vi "Read As File_Sync.vi"(7 "mode (OpenOrCreate)":i32(ring)=4 items=["CreateNew"=1, "Create"=2, "Open"=3, "OpenOrCreate"=4, "Truncate"=5, "Append"=6], 8 "error in (no error)":errorcluster, 10 "FilePath":path, 11 "HttpContent in":refnum<class "HttpContent.lvclass">) -> (0 "error out":errorcluster, 1 "IsCompleted":bool, 2 "FilePath (dup)":path, 3 "HttpContent out":refnum<class "HttpContent.lvclass">, 4 "Canceled":bool)   [LabVIEW 2018, in "HttpClient_NET.lvlib" / "HttpContent.lvclass"]
doc: "<b> </b> <b> </b>\nHttpClient_NET\nJustin Young - Viviota\nCopyright (c) 2021\nLicense: BSD"
uses:
  HttpContent.lvclass
  Types/HttpNet_error_enum.ctl
  HttpClient_NET.lvlib
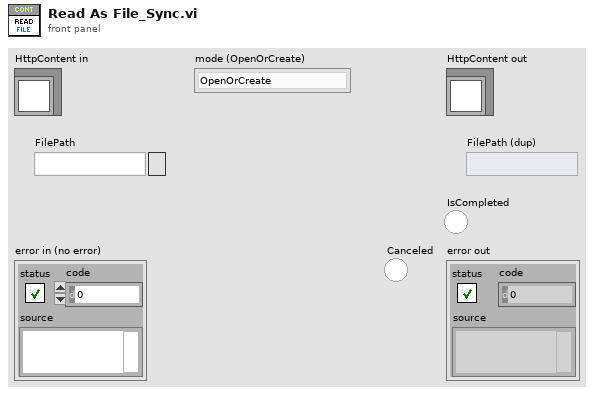
[diagram p1: front panel]
types:
  T1 = typedef "HttpClient_NET.lvlib/HttpNet_error_enum.ctl" = enum16{"REST method is not available", "URL cannot be blank", "Output filepath cannot be empty", "Input filepath cannot be empty", "Internal .NET error %s", "Output filepath cannot be directory", "Download Task no longer exists", "Mutipart Put not supported from REST Client Interface.  Please revert to lower level classes"}
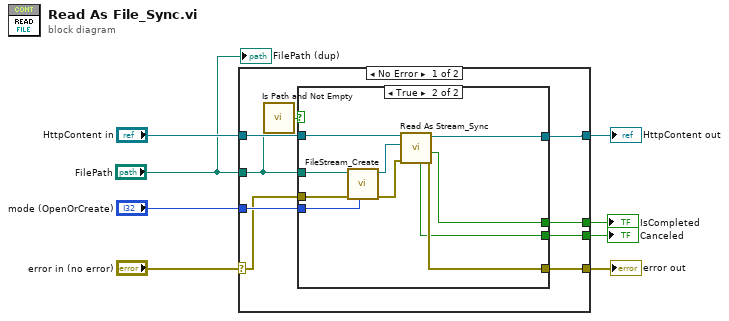
[diagram p0: block diagram]
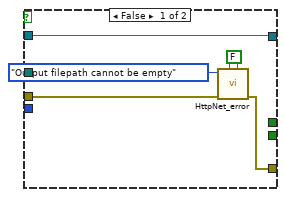
[diagram p2: hidden frame]
diagram:
  n1 = case shown="No Error" "error in (no error)" {
    selector: "error in (no error)" -> [w13 w34]
    tunnel: [w14 w34] -> w7
    tunnel: [w16 w33] -> w5
    tunnel: "HttpContent in" -> [w17 w33]
    tunnel: "mode (OpenOrCreate)" -> [w15 _]
    tunnel: "FilePath" -> [w10 _]
    tunnel: [w12 _] -> w2
    tunnel: [w11 _] -> w1
    frame No Error {
      n2 = call <vilib>:"Is Path and Not Empty.vi"("path"=w10) -> ("Is Path and Not Empty?"=w9:bool)  [unwired: 4 in]
      n3 = case shown="True" w9 {
        tunnel: w17 -> [w22 w32]
        tunnel: [w22 w31] -> w16
        tunnel: w15 -> [_ w25]
        tunnel: [w20 w28] -> w14
        tunnel: w13 -> [w21 w27]
        tunnel: [_ w23] -> w12
        tunnel: [_ w24] -> w11
        tunnel: w10 -> [_ w26]
        frame False {
          w18 = FALSE ("OverrideExistingErrors [T]")
          n4 = call "HttpNet_error.vi"("ShowCallChain [T]"=w18, "OverrideExistingErrors [T]"=w18, "Error In"=w21, "Error"=HttpNet_error_enum."Output filepath cannot be empty") -> ("Error Out"=w20:errorcluster)  [unwired: 7 in]
        }
        frame True {
          n5 = call "FileStream_Create.vi"("mode [OpenOrCreate]"=w25, "error in (no error)"=w27, "FilePath"=w26) -> ("error out"=w29:errorcluster, "FileStream"=w30:refnum<k24>)  [unwired: 7 in]
          n6 = call "Read As Stream_Sync.vi"("error in (no error)"=w29, "stream"=w30, "HttpContent in"=w32) -> ("error out"=w28:errorcluster, "IsCompleted"=w24:bool, "HttpContent out"=w31:refnum<class "HttpContent.lvclass">, "Canceled"=w23:bool)  [unwired: 5 in]
        }
      }
    }
    frame Error {
    }
  }
  "error out" <- w7
  "HttpContent out" <- w5
  "Canceled" <- w2
  "IsCompleted" <- w1
  "FilePath (dup)" <- "FilePath"
